vi "禹山电导率_获取用户校准参数.vi"(8 "error in (no error)":errorcluster caption="错误输入（无错误）", 11 "MB_Serial session in":refnum<class "MB_Master_Serial.lvclass">) -> (0 "error out":errorcluster caption="错误输出", 2 "输出值":cluster{"K":sgl, "B":sgl}, 3 "MB_Serial session out":refnum<class "MB_Master_Serial.lvclass">)   [LabVIEW 2016, in "斯坦道多参数.lvlib"]
uses:
  <vilib>/Plasmionique/MB Master/MB_Master_Serial/MB_Master_Serial.lvclass
  C:/Program Files (x86)/National Instruments/LabVIEW 2016/vi.lib/Plasmionique/MB Master/MB_Master/MB_Master.lvclass
  <vilib>/Plasmionique/MB Master/MB Master.lvlib
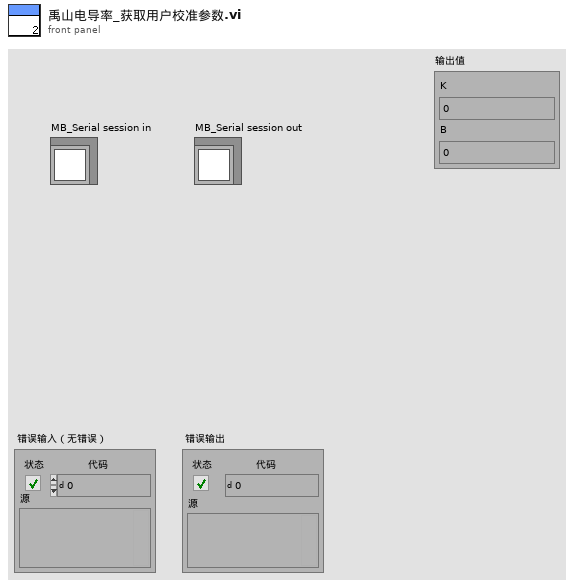
[diagram p1: front panel]
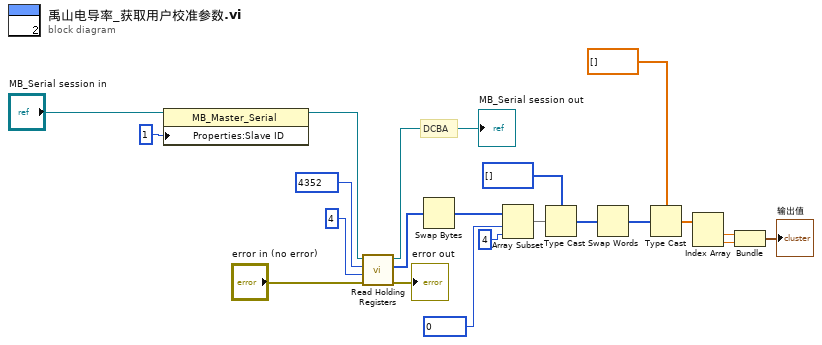
[diagram p0: block diagram]
diagram:
  # "DCBA"
  n1 = property class="MB_Master_Serial"(reference="MB_Serial session in", "Properties:Slave ID"=u16 1 ("y")) -> (reference out=w8:refnum<class "MB_Master_Serial.lvclass">)  [unwired: 1 in, 1 out]
  n2 = call <vilib>:"Read Holding Registers.vi"("error in (no error)"="error in (no error)", "quantity"=u16 4, "starting address"=u16 4352, "MB session in"=w8) -> ("error out"=→"error out":errorcluster, "Registers"=w4:u16[], "MB session out"=→"MB_Serial session out":refnum<class "MB_Master_Serial.lvclass">)  [unwired: 5 in]
  n3 = Swap Bytes(anything=w4) -> (byte swapped=w3:u16[])
  n4 = Array Subset(array=w3, index=u16 0 ("starting address"), length=4 ("长度")) -> (w2:u16[])
  n5 = Type Cast(type=u32[] [] ("数组 2"), x=w2) -> (*(type *) &x=w15:u32[])
  n6 = Swap Words(1:w15) -> (0:w17:u32[])
  n7 = Type Cast(type=sgl[] [] ("数组 2"), x=w17) -> (*(type *) &x=w13:sgl[])
  n8 = Index Array(array=w13) -> (element #1=w12:sgl, element #2=w11:sgl)  [unwired: 2 in]
  n9 = Bundle("数值"=w12, "数值"=w11) -> (→"输出值":cluster{"数值":sgl, "数值":sgl})  [unwired: 1 in]
